vi "yolov5_demo.vi"() -> ()   [LabVIEW 2021]
uses:
  bin/detect_lay.dll
panel:
  out "output":i32[](array[numeric])
  out "error out 2":errorcluster
  out "error out":errorcluster
  out "time(ms)":dbl
  in  "img_Path":path
  out "roi":T1(plugin-control)
  out "Original":T1(plugin-control)
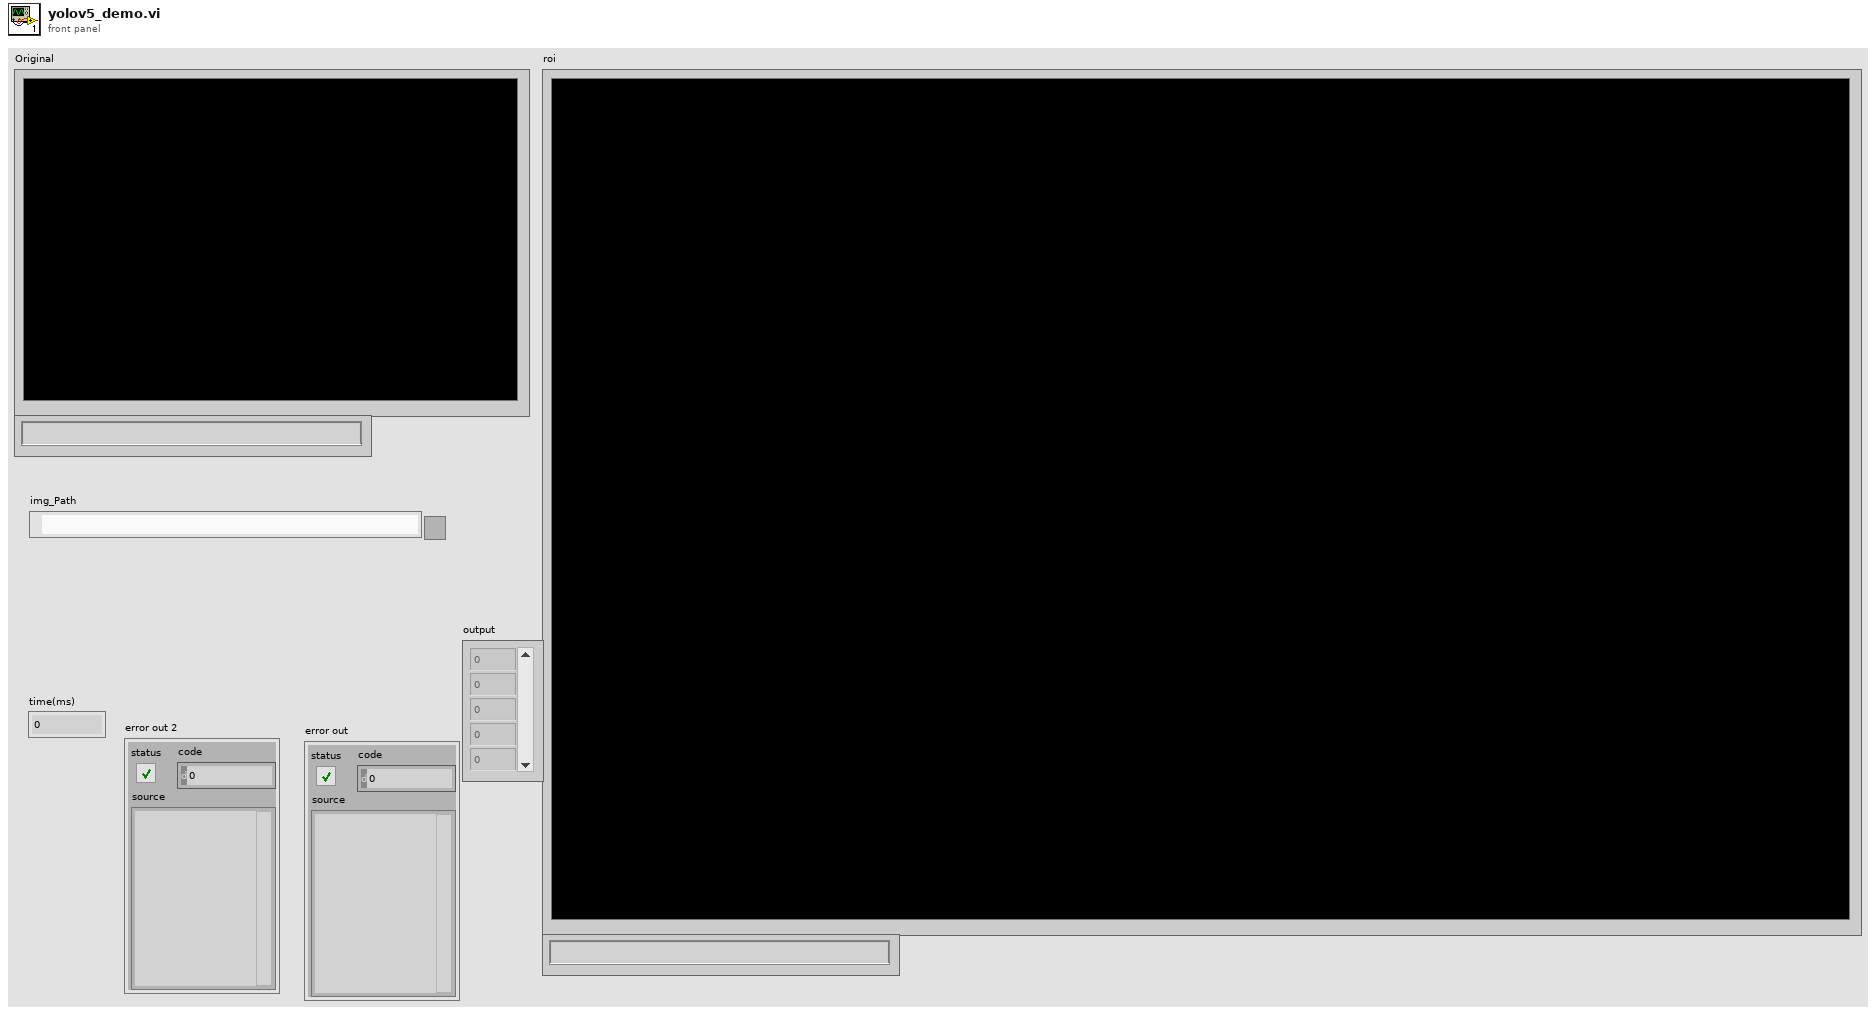
[diagram p1: front panel]
types:
  T1 = typedef "IMAQ Image.ctl" = refnum<image>
  T2 = typedef "Image Type" = u32
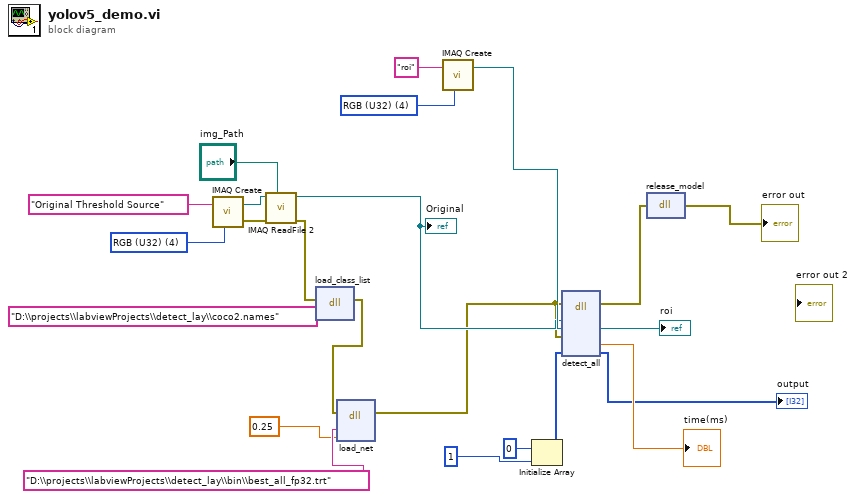
[diagram p0: block diagram]
diagram:
  w16 = T2 4 items=["Grayscale (U8)", "Grayscale (I16)", "Grayscale (SGL)", "Complex (CSG)", "RGB (U32)", "HSL (U32)", "RGB (U64)", "Grayscale (U16)"] ("Image Type")
  w20 = T2 4 items=["Grayscale (U8)", "Grayscale (I16)", "Grayscale (SGL)", "Complex (CSG)", "RGB (U32)", "HSL (U32)", "RGB (U64)", "Grayscale (U16)"] ("Image Type")
  n1 = call "IMAQ Create"("Image Name"="Original Threshold Source", "Image Type"=w20) -> ("New Image"=w22:T1, "error out"=w21:errorcluster)  [unwired: 3 in]
  n2 = call "IMAQ ReadFile 2"("File Path"="img_Path", "error in (no error)"=w21, "Image"=w22) -> ("error out"=w12:errorcluster, "Image Out"=w14:T1)  [unwired: 4 in, 3 out]
  "Original" <- w14
  n3 = dll-call lib="D:/projects/labviewProjects/detect_lay/bin/detect_lay.dll" fn="load_class_list"(error in=w12, "path"="D:\\projects\\labviewProjects\\detect_lay\\coco2.names") -> (error out=w13:errorcluster)  [unwired: 4 in, 1 out]
  n4 = dll-call lib="D:/projects/labviewProjects/detect_lay/bin/detect_lay.dll" fn="load_net"(error in=w13, "path"="D:\\projects\\labviewProjects\\detect_lay\\bin\\best_all_fp32.trt", "score_threshold"=0.25) -> (error out=w9:errorcluster)  [unwired: 5 in, 1 out]
  n5 = call "IMAQ Create"("Image Name"="roi", "Image Type"=w16) -> ("New Image"=w15:T1)  [unwired: 3 in, 1 out]
  n6 = Initialize Array(0, 1) -> (w2:i32[])
  n7 = dll-call lib="D:/projects/labviewProjects/detect_lay/bin/detect_lay.dll" fn="detect_all"(error in=w9, "sourceHandle_src"=w14, "destHandle"=w15, "errorHandle"=w9, "exist"=w2) -> (error out=w6:errorcluster, "destHandle"=→"roi":T1, "time"=→"time(ms)":dbl, "exist"=→"output":i32[])  [unwired: 6 in, 1 out]
  n8 = dll-call lib="D:/projects/labviewProjects/detect_lay/bin/detect_lay.dll" fn="release_model"(error in=w6) -> (error out=→"error out":errorcluster)  [unwired: 3 in, 1 out]
